vi "Read Module Menu Name.vi"(8 "error in":errorcluster, 11 "EthernetIP editor node in":refnum<class "EIP Tag API editor node.lvclass">) -> (0 "error out":errorcluster, 2 "Menu Name":string, 3 "EthernetIP editor node out":refnum<class "EIP Tag API editor node.lvclass">)   [LabVIEW 2013, in "EIP Tag API editor node.lvclass"]
uses:
  EIP Tag API editor node.lvclass
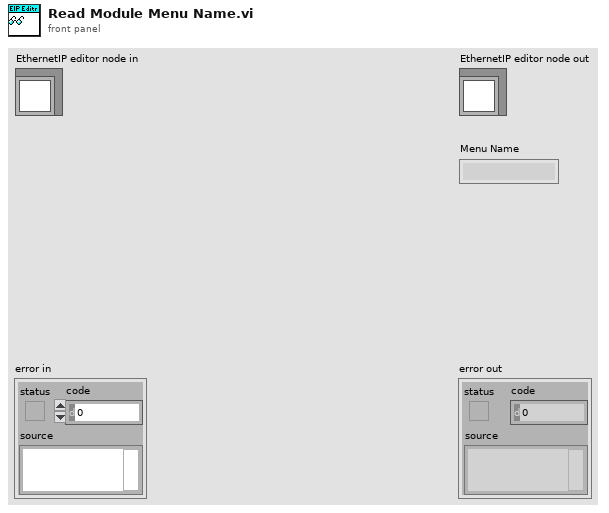
[diagram p1: front panel]
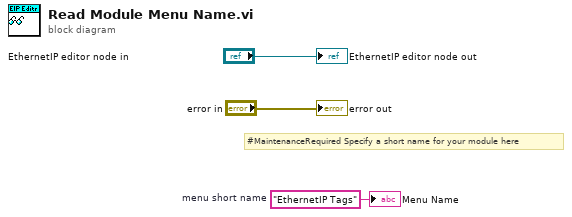
[diagram p0: block diagram]
diagram:
  w1 = "EthernetIP Tags"  # menu short name
  # "#MaintenanceRequired Specify a short name for your module here"
  "error out" <- "error in"
  "EthernetIP editor node out" <- "EthernetIP editor node in"
  "Menu Name" <- w1
